vi "Write json to AI DB one.vi"(7 "conninfo":T1={"host"="localhost", "port"="5432", "client_encoding"="WIN1251", "dbname"="system", "user"="postgres", "password"=""}, 8 "error in (no error)":errorcluster, 10 "JSON Data In":string, 11 "AI in":T2) -> (0 "error out":errorcluster, 3 "AI out":T2)   [LabVIEW 2019, in "Inputs.lvlib"]
doc: "sorting to fcode_full column\nfa_1 request returns fcode_full without ltree points GM1QN3_XQ01\nfa_3 request returns fcode_full with ltree points GM1.QN3_XQ01\n {\"GM1QN3_XQ01\":{\"instrument_gain\":10,\n \"input_register_min\":6554,\n \"input_register_max\":32767,\n \"input_pv_max\":2.5},\n \"GM1QN4_XQ01\":{\"instrument_gain\":10,\n \"input_register_min\":6554,\n \"input_register_max\":32767,\n \"input_pv_max\":4.99}\n}"
uses:
  Inputs.lvlib
  Ctl/AI.ctl
  Ctl/AI short.ctl
  Ctl/Parameter State.ctl
  Database/ctl/Coninfo.ctl
  Database/PostgreSQL2LabVIEW/libpqUtility/src/PQexecute.vi
  Database/PostgreSQL2LabVIEW/libpqUtility/src/PQconnect.vi
  Database/PostgreSQL2LabVIEW/libpqUtility/src/PQclose.vi
  <vilib>/JDP Science/JSONtext/Find Multiple Items.vi
  Database/PostgreSQL2LabVIEW/libpqlv/src/PQresultErrorMessage.vi
  Database/PostgreSQL2LabVIEW/libpqUtility/src/PQclear.vi
  Database/PostgreSQL2LabVIEW/libpqlv/src/PQsendQuery.vi
  Database/PostgreSQL2LabVIEW/libpqlv/src/PQgetResult.vi
  Database/PostgreSQL2LabVIEW/libpqlv/src/PQresultStatus.vi
  Database/PostgreSQL2LabVIEW/libpqlv/src/PQfinish.vi
  Database/PostgreSQL2LabVIEW/libpqlv/src/PQconnectdb.vi
  Database/PostgreSQL2LabVIEW/libpqlv/src/PQerrorMessage.vi
  Database/PostgreSQL2LabVIEW/libpqlv/src/PQstatus.vi
  <vilib>/dlg_ctls.llb/Space Constant.vi
  <vilib>/JDP Science/JSONtext/String Subset.vi
  <vilib>/JDP Science/JSONtext/support/Strip Quotes and Unescape.vi
  Database/PostgreSQL2LabVIEW/libpqlv/src/PQclear.vi
  <vilib>/JDP Science/JSONtext/support/Unescape JSON string.vi
  <vilib>/JDP Science/JSONtext/Parsing/Parse Full Path or Item Name.vi
  <vilib>/JDP Science/JSONtext/Offset/Find Item Locations by Path.vi
  <vilib>/JDP Science/JSONtext/Get Array Elements.vi
  Userlib.lvlib
  Database/PostgreSQL.lvlib
panel:
  # "Analog parameters"
  # "Description of analog parameters"
  # "Analog parameters"
  # "Description of analog parameters"
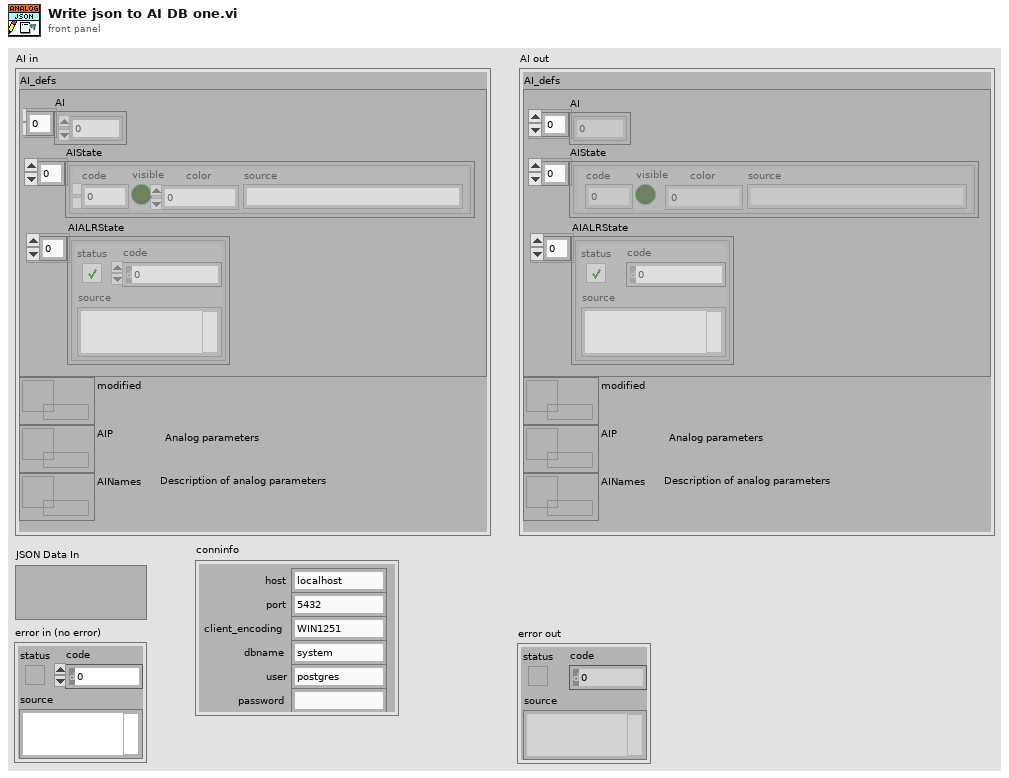
[diagram p1: front panel]
types:
  T1 = typedef "PostgreSQL.lvlib/Coninfo.ctl" = cluster{"host":string, "port":string, "client_encoding":string, "dbname":string, "user":string, "password":string}
  T2 = typedef "Inputs.lvlib/AI.ctl" = cluster{"AI_defs":T3, "modified":refnum<data-value>, "AIP":refnum<data-value>, "AINames":refnum<data-value>}
  T3 = typedef "Inputs.lvlib/AI short.ctl" = cluster{"AI":dbl[], "AIState":T4[], "AIALRState":errorcluster[]}
  T4 = typedef "Inputs.lvlib/Parameter State.ctl" = cluster{"code":i32, "visible":bool, "color":u32, "source":string}
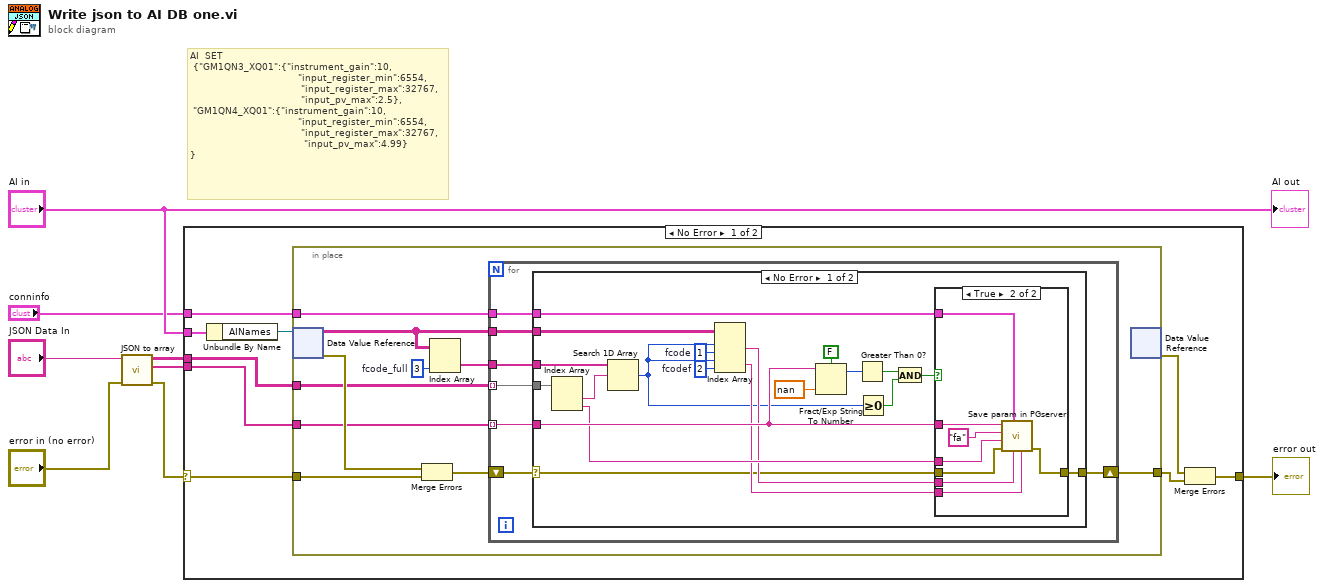
[diagram p0: block diagram]
diagram:
  # "AI  SET\n {\"GM1QN3_XQ01\":{\"instrument_gain\":10,\n                                    \"input_register_min\":6554,\n                                     \"input_register_max\":32767,\n                                     \"input_pv_max\":2.5},\n \"GM1QN4_XQ01\":{\"instrument_gain\":10,\n                                    \"input_register_min\":6554,\n                                     \"input_register_max\":32767,\n                                      \"input_pv_max\":4.99}\n}"
  n1 = call "JSON to array.vi"("error in (no error)"="error in (no error)", "JSON Data In"="JSON Data In") -> ("error out"=w5:errorcluster, "values"=w2:string[], "names"=w3:string[][])  [unwired: 7 in]
  n2 = case shown="No Error" w5 {
    selector: w5 -> [w12 w65]
    tunnel: [w16 w65] -> w8
    tunnel: "AI in" -> [w17 _]
    tunnel: w2 -> [w11 _]
    tunnel: w3 -> [w14 _]
    tunnel: "conninfo" -> [w13 _]
    frame No Error {
      n3 = Unbundle By Name(w17) -> ("AINames"=w15:refnum<data-value>)
      n4 = in-place {
        in-place-border: w11 -> [w25]
        in-place-border: [w26] -> w9
        in-place-border: w14 -> [w23]
        in-place-border: w12 -> [w21]
        in-place-border: w13 -> [w20]
        w18 = 3  # fcode_full
        n5 = in-place-dvr #1(w15) -> (w19:string[][], w27:errorcluster)
        n6 = Merge Errors(w27, w21) -> (w24:errorcluster)
        n7 = Index Array(array=w19, index (col)=w18) -> (element=w22:string[])  [unwired: 1 in]
        n8 = for {
          tunnel: w19 -> [w30]
          tunnel: w25 -> [w29] mode=indexing
          shift-right: [w34] -> w26
          shift-left: w24 -> [w28]
          tunnel: w23 -> [w33] mode=indexing
          tunnel: w22 -> [w32]
          tunnel: w20 -> [w31]
          n9 = case shown="No Error" w28 {
            selector: w28 -> [w44 w64]
            tunnel: [w42 w64] -> w34
            tunnel: w33 -> [w54 _]
            tunnel: w32 -> [w52 _]
            tunnel: w31 -> [w43 _]
            tunnel: w30 -> [w51 _]
            tunnel: w29 -> [w48 _]
            frame No Error {
              w35 = 2  # fcodef
              w36 = 1  # fcode
              n10 = Index Array(array=w54) -> (element #1=w53:string, element #2=w47:string)  [unwired: 2 in]
              n11 = Search 1D Array(1D array=w52, element=w53) -> (index of element=w40:i32)  [unwired: 1 in]
              n12 = Index Array(array=w51, index (row) #1=w40, index (col) #1=w36, index (row) #2=w40, index (col) #2=w35) -> (element #1=w46:string, element #2=w45:string)
              n13 = Fract/Exp String To Number(use system decimal point (T)=FALSE, string=w48, default (0 dbl)=nan) -> (offset past number=w41:i32)  [unwired: 1 in, 1 out]
              n14 = Greater Than 0?(x=w41) -> (x > 0?=w39:bool)
              n15 = Greater Or Equal To 0?(x=w40) -> (x >= 0?=w38:bool)
              n16 = And(x=w39, y=w38) -> (x .and. y?=w37:bool)
              n17 = case shown="True" w37 {
                tunnel: w48 -> [_ w56]
                tunnel: w47 -> [_ w63]
                tunnel: w46 -> [_ w62]
                tunnel: w45 -> [_ w61]
                tunnel: w44 -> [w55 w60]
                tunnel: w43 -> [_ w59]
                tunnel: [w55 w58] -> w42
                frame False {
                  # "Not number"
                }
                frame True {
                  n18 = call "Save param in PGserver.vi"("Param row name 2"=w61, "Param row name1"=w62, "conninfo"=w59, "error in (no error)"=w60, "Param column Name"=w63, "Param Table"="fa", "Parameter"=w56) -> ("error out"=w58:errorcluster)  [unwired: 4 in]
                }
              }
            }
            frame Error {
            }
          }
        }
        n19 = in-place-dvr #1() -> (w10:errorcluster)  [unwired: 1 in, 1 out]
      }
      n20 = Merge Errors(w10, w9) -> (w16:errorcluster)
    }
    frame Error {
    }
  }
  "error out" <- w8
  "AI out" <- "AI in"
